vi "AlazarGetTriggerAddress.vi"(0 "Handle":u64, 1 "Record":u32, 5 "error in (no error)":errorcluster) -> (14 "Handle":u64, 15 "Trigger Address":u32, 16 "Timestamp High Part":u32, 17 "Timestamp Low Part":u32, 18 "Return Code":u32, 19 "error out":errorcluster)   [LabVIEW 2018]
doc: "Get the timestamp and trigger address of the trigger event in a record acquired to on-board memory."
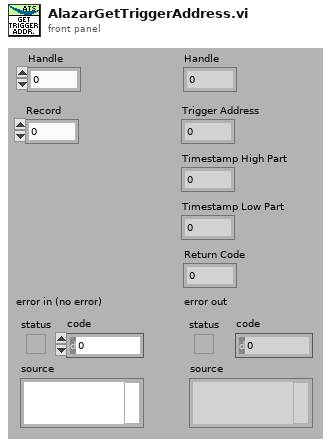
[diagram p1: front panel]
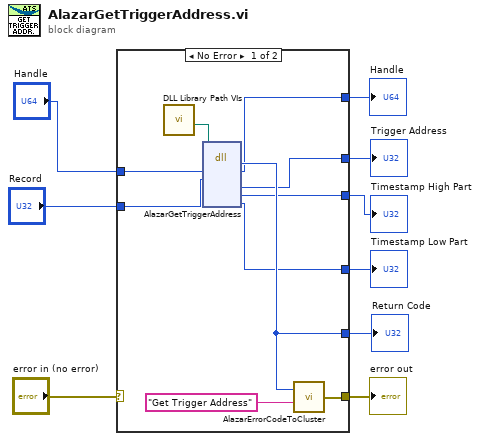
[diagram p0: block diagram]
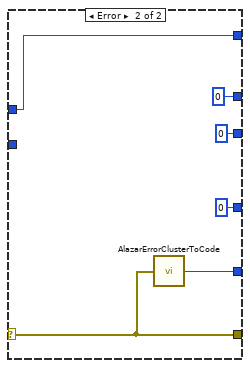
[diagram p2: hidden frame]
diagram:
  n1 = case shown="No Error" "error in (no error)" {
    selector: "error in (no error)" -> [_ w25]
    tunnel: [w16 w25] -> w8
    tunnel: "Handle" -> [w19 w23]
    tunnel: [w15 w23] -> w6
    tunnel: [w18 w24] -> w5
    tunnel: [w14 u32 0] -> w4
    tunnel: [w13 u32 0] -> w3
    tunnel: [w12 u32 0] -> w2
    tunnel: "Record" -> [w11 _]
    frame No Error {
      n2 = call "DLL Library Path VIs.vi"() -> ("Alazar"=w10:path)  [unwired: 9 in, 2 out]
      n3 = dll-call lib="C:/Project/SerialSectOCT - FFT GPU/SerialSectOCT/Labview Software/DLL/ATSApi.dll" fn="AlazarGetTriggerAddress"(path in=w10, "handle"=w19, "record"=w11) -> ("return type"=w18:u32, "handle"=w15:u64, "triggerAddress"=w12:u32, "timestampHighPart"=w13:u32, "timestampLowPart"=w14:u32)  [unwired: 6 in, 2 out]
      n4 = call "AlazarErrorCodeToCluster.vi"("Message"="Get Trigger Address", "Error Code"=w18) -> ("error out"=w16:errorcluster)
    }
    frame Error {
      n5 = call "AlazarErrorClusterToCode.vi"("error in (no error)"=w25) -> ("Error Code"=w24:u32)
    }
  }
  "Handle" <- w6
  "error out" <- w8
  "Return Code" <- w5
  "Trigger Address" <- w2
  "Timestamp High Part" <- w3
  "Timestamp Low Part" <- w4
